vi "Shooter Global.vi"() -> ()   [LabVIEW 2019]
panel:
  in  "Motor Power":dbl
  in  "Requested RPM":dbl
  in  "Current RPM":dbl
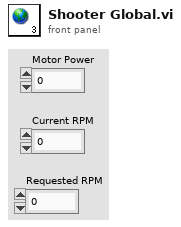
[diagram p1: front panel]
diagram:
